vi "DHE_Aliases2.vi"(5 "expand reg":bool, 7 "action":T2(ring)=enum."find", 10 "name in":string) -> (1 "found?":bool, 2 "name out":string, 4 "register?":bool)   [LabVIEW 2016]
uses:
  private/vis/DHE_alias.ctl
  <vilib>/Utility/config.llb/Read Key (String).vi
  <vilib>/Utility/config.llb/NI_LVConfig.lvlib
panel:
  out "aliases":T1[](array[typedef])
  in  "alias":T1
  in  "error in (no error)":errorcluster
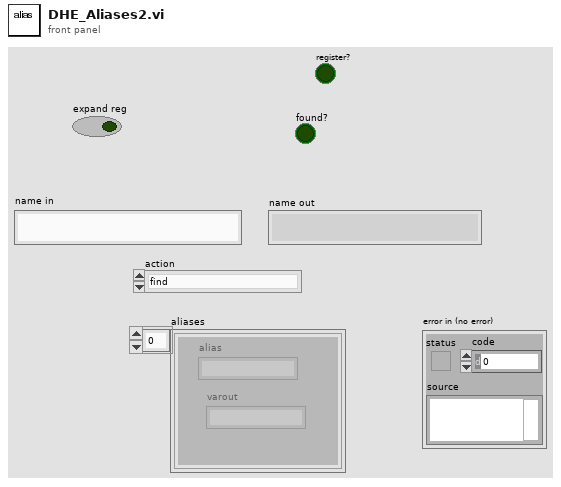
[diagram p1: front panel]
types:
  T1 = typedef "DHE_alias.ctl" = cluster{"alias":string, "varout":string}
  T2 = enum16{"read from file", "find", "get", "add", "delete", "clear "}
  T3 = typedef "NI_LVConfig.lvlib/Config Data RefNum.ctl" = refnum<k1>
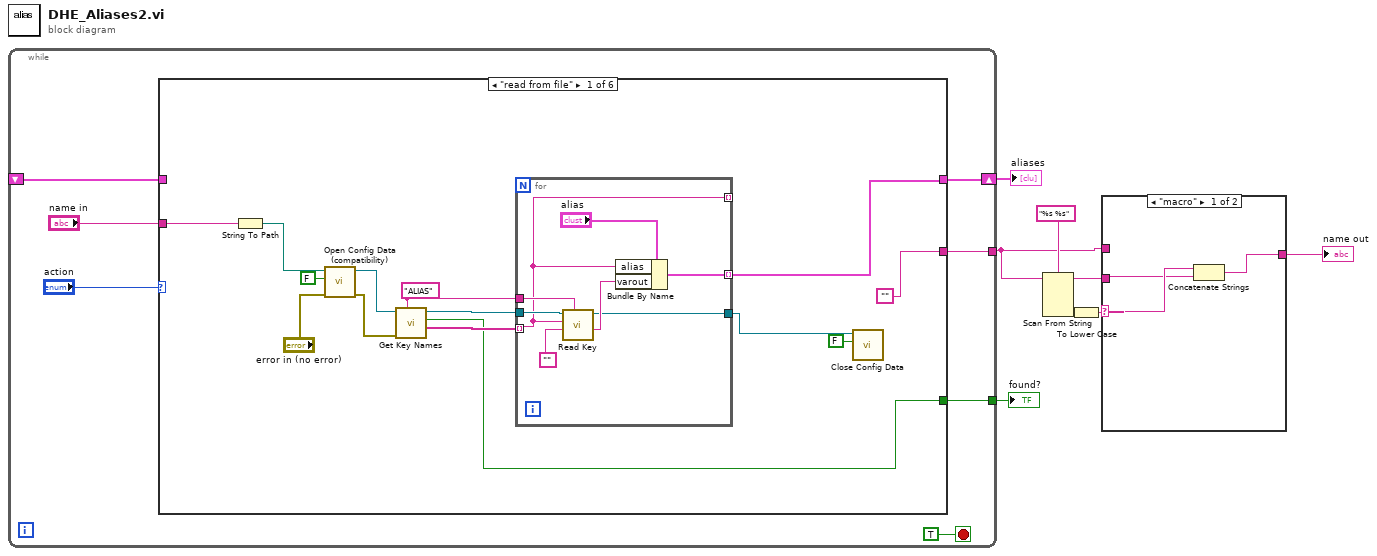
[diagram p0: block diagram]
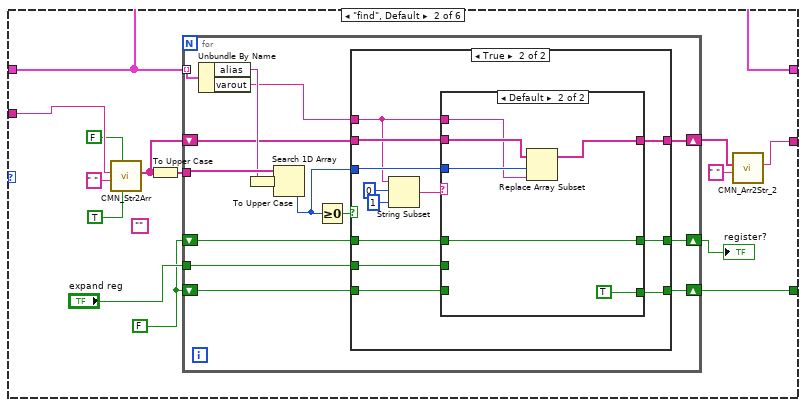
[diagram p3: hidden frame]
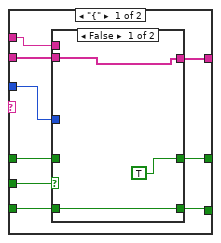
[diagram p5: hidden frame]
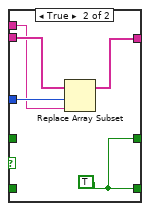
[diagram p6: hidden frame]
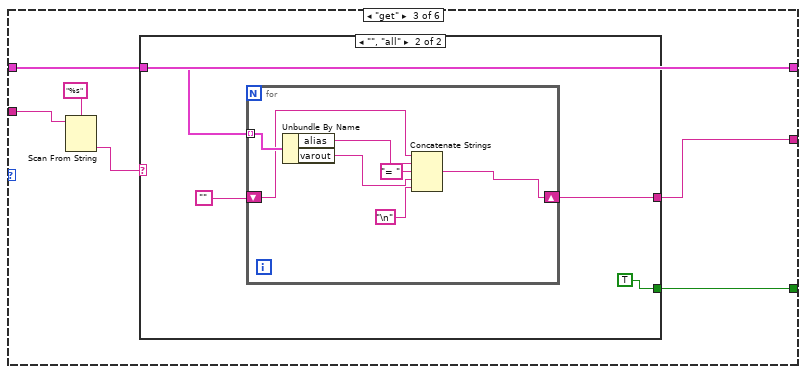
[diagram p7: hidden frame]
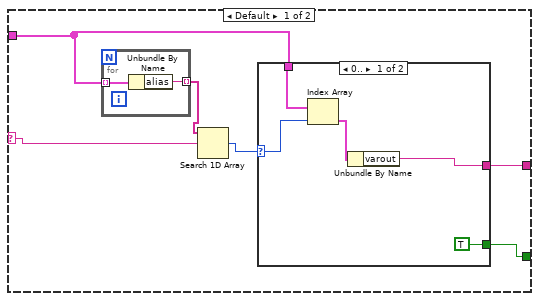
[diagram p8: hidden frame]
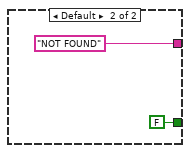
[diagram p9: hidden frame]
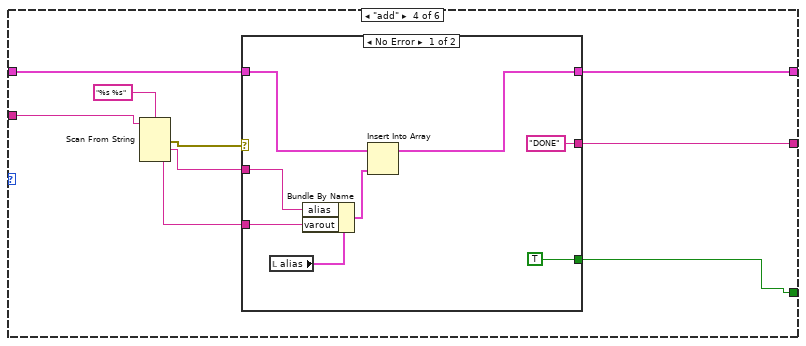
[diagram p10: hidden frame]
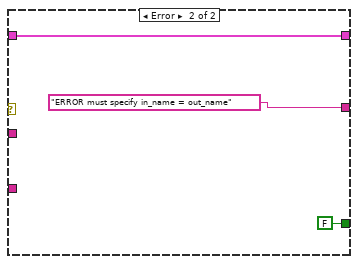
[diagram p11: hidden frame]
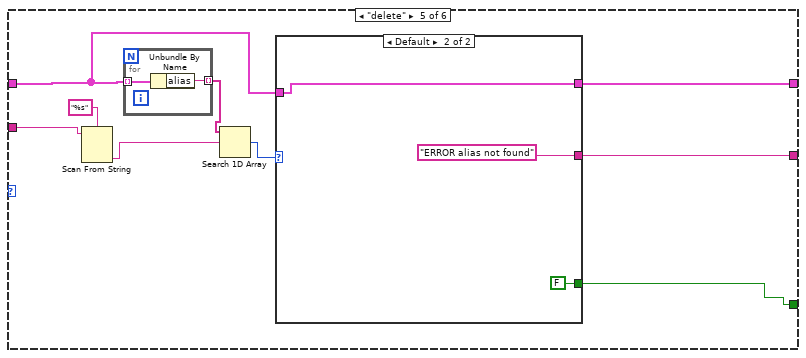
[diagram p12: hidden frame]
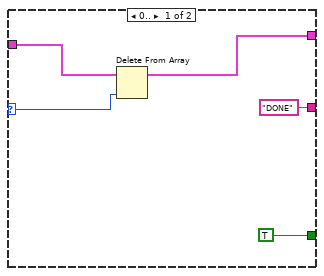
[diagram p13: hidden frame]
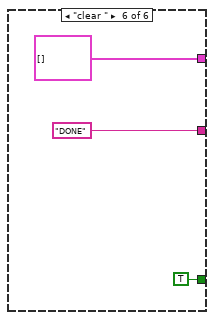
[diagram p14: hidden frame]
diagram:
  n1 = while {
    shift-right: [w14] -> w8
    shift-left: _ -> [w13]
    tunnel: [w10] -> w2
    tunnel: [w9] -> w7
    stop <- TRUE stop-if-true
    n2 = case shown="\"read from file\"" "action" {
      tunnel: [w23 w51 w109 w138 w162 T1[] []] -> w14
      tunnel: w13 -> [_ w51 w109 w144 w157 _]
      tunnel: "name in" -> [w21 w50 w107 w143 w164 _]
      tunnel: ["" w43 w108 w137 w161 "DONE" ("string out")] -> w10
      tunnel: [w16 w41 w104 w136 w156 TRUE ("section exists?")] -> w9
      frame "read from file" {
        w29 = "ALIAS" ("section")
        n3 = String To Path(string=w21) -> (path=w20:path)
        n4 = call <vilib>:"Open Config Data (compatibility).vi"("error in (no error)"="error in (no error)", "create file if necessary (T)"=FALSE, "configuration file path"=w20) -> ("error out"=w25:errorcluster, "refnum"=w24:T3)  [unwired: 6 in, 1 out]
        n5 = call <vilib>:"Get Key Names.vi"("section"=w29, "error in (no error)"=w25, "refnum"=w24) -> ("key names"=w28:string[], "section exists?"=w16:bool, "refnum out"=w27:T3)  [unwired: 6 out]
        n6 = for {
          tunnel: w27 -> [w37]
          tunnel: w29 -> [w36]
          tunnel: w28 -> [w31] mode=indexing
          tunnel: [w32] -> w23 mode=indexing
          tunnel: [w31] -> _ mode=indexing
          tunnel: [w30] -> w18
          n7 = call-poly <vilib>:"Read Key.vi"("section"=w36, "default value"="", "key"=w31, "refnum"=w37) -> ("value"=w33:string, "refnum out"=w30:T3)  [unwired: 2 in, 4 out]
          n8 = Bundle By Name(cluster="alias", "alias"=w31, "varout"=w33) -> (w32:T1)
        }
        n9 = call <vilib>:"Close Config Data.vi"("write file if changed (T)"=FALSE, "refnum"=w18) -> ()  [unwired: 8 in, 2 out]
      }
      frame "find", Default {
        w40 = FALSE
        (unwired) ""
        n10 = call "CMN_Str2Arr.vi"("trim"=TRUE, "strip quotation marks"=FALSE, "separator"=" ", "string in"=w50) -> ("Array out"=w46:string[])  [unwired: 7 in]
        n11 = To Upper Case(1:w46) -> (0:w38:string[])
        n12 = for {
          tunnel: w51 -> [w65] mode=indexing
          tunnel: w38 -> [w64]
          shift-right: [w58] -> w45
          shift-left: w46 -> [w61]
          tunnel: "expand reg" -> [w57]
          shift-right: [w55] -> w41
          shift-left: w40 -> [w56]
          shift-right: [w53] -> w39
          shift-left: w40 -> [w54]
          n13 = Unbundle By Name(w65) -> ("alias"=w63:string, "varout"=w59:string)
          n14 = To Upper Case(1:w63) -> (0:w52:string)
          n15 = Search 1D Array(1D array=w64, element=w52) -> (index of element=w60:i32)  [unwired: 1 in]
          n16 = Greater Or Equal To 0?(x=w60) -> (x >= 0?=w62:bool)
          n17 = case shown="True" w62 {
            tunnel: w61 -> [w68 w80]
            tunnel: w60 -> [_ w79]
            tunnel: w59 -> [_ w77]
            tunnel: [w68 w78] -> w58
            tunnel: w57 -> [_ w73]
            tunnel: w56 -> [w67 w72]
            tunnel: [w67 w71] -> w55
            tunnel: w54 -> [w66 w70]
            tunnel: [w66 w69] -> w53
            frame False {
            }
            frame True {
              n18 = String Subset(string=w77, offset (0)=0, length (rest)=1 ("length (rest)")) -> (substring=w74:string)
              n19 = case shown="Default" w74 {
                tunnel: w80 -> [w88 w103]
                tunnel: w79 -> [w87 w102]
                tunnel: w77 -> [w86 w101]
                tunnel: [w85 w100] -> w78
                tunnel: w73 -> [w89 _]
                tunnel: w72 -> [w84 _]
                tunnel: [w83 TRUE] -> w71
                tunnel: w70 -> [w82 w98]
                tunnel: [w81 w98] -> w69
                frame "{" {
                  n20 = case shown="False" w89 {
                    tunnel: w88 -> [w92 w96]
                    tunnel: w87 -> [_ w97]
                    tunnel: w86 -> [_ w95]
                    tunnel: [w92 w94] -> w85
                    tunnel: w84 -> [w91 _]
                    tunnel: [w91 w93] -> w83
                    tunnel: w82 -> [_ _]
                    tunnel: [TRUE w93] -> w81
                    frame False {
                    }
                    frame True {
                      w93 = TRUE
                      n21 = Replace Array Subset(array=w96, new element=w95, index=w97) -> (w94:string[])
                    }
                  }
                }
                frame Default {
                  n22 = Replace Array Subset(array=w103, new element=w101, index=w102) -> (w100:string[])
                }
              }
            }
          }
        }
        "register?" <- w39
        n23 = call "CMN_Arr2Str_2.vi"("separator"=" ", "Array in"=w45) -> ("string out"=w43:string)  [unwired: 9 in]
      }
      frame "get" {
        n24 = Scan From String(format string="%s", input string=w107) -> (output 1=w105:string)  [unwired: 3 in, 3 out]
        n25 = case shown="\"\", \"all\"" w105 {
          selector: w105 -> [w114 _]
          tunnel: w109 -> [w112 w128]
          tunnel: [w111 w126] -> w108
          tunnel: [w110 TRUE ("section exists?")] -> w104
          frame Default {
            n26 = for {
              tunnel: w112 -> [w124] mode=indexing
              tunnel: [w123] -> w115 mode=indexing
              n27 = Unbundle By Name(w124) -> ("alias"=w123:string)
            }
            n28 = Search 1D Array(1D array=w115, element=w114) -> (index of element=w113:i32)  [unwired: 1 in]
            n29 = case shown="0.." w113 {
              selector: w113 -> [w119 _]
              tunnel: w112 -> [w120 _]
              tunnel: [w117 "NOT FOUND" ("varout")] -> w111
              tunnel: [TRUE ("section exists?") FALSE ("section exists?")] -> w110
              frame 0.. {
                n30 = Index Array(array=w120, index=w119) -> (element=w118:T1)
                n31 = Unbundle By Name(w118) -> ("varout"=w117:string)
              }
              frame Default {
              }
            }
          }
          frame "", "all" {
            n32 = for {
              tunnel: w128 -> [w135] mode=indexing
              shift-right: [w129] -> w126
              shift-left: "" -> [w130]
              n33 = Unbundle By Name(w135) -> ("alias"=w134:string, "varout"=w132:string)
              n34 = Concatenate Strings(w130, w134, "= " ("string"), w132, "\n") -> (w129:string)
            }
          }
        }
      }
      frame "add" {
        n35 = Scan From String(format string="%s %s", input string=w143) -> (error out=w141:errorcluster, output 1=w140:string, output 2=w139:string)  [unwired: 4 in, 2 out]
        n36 = case shown="No Error" w141 {
          tunnel: w144 -> [w152 w155]
          tunnel: w140 -> [w150 _]
          tunnel: w139 -> [w149 _]
          tunnel: [w147 w155] -> w138
          tunnel: ["DONE" ("string out") "ERROR must specify in_name = out_name" ("string out")] -> w137
          tunnel: [TRUE ("section exists?") FALSE ("section exists?")] -> w136
          frame No Error {
            n37 = local read "alias"() -> (w151:T1)
            n38 = Bundle By Name(cluster=w151, "alias"=w150, "varout"=w149) -> (w148:T1)
            n39 = Insert Into Array(array=w152, new element=w148) -> (w147:T1[])  [unwired: 1 in]
          }
          frame Error {
          }
        }
      }
      frame "delete" {
        n40 = Scan From String(format string="%s", input string=w164) -> (output 1=w159:string)  [unwired: 3 in, 3 out]
        n41 = for {
          tunnel: w157 -> [w166] mode=indexing
          tunnel: [w165] -> w160 mode=indexing
          n42 = Unbundle By Name(w166) -> ("alias"=w165:string)
        }
        n43 = Search 1D Array(1D array=w160, element=w159) -> (index of element=w158:i32)  [unwired: 1 in]
        n44 = case shown="Default" w158 {
          selector: w158 -> [w169 _]
          tunnel: [w168 w173] -> w162
          tunnel: ["DONE" ("string out") "ERROR alias not found" ("string out")] -> w161
          tunnel: w157 -> [w170 w173]
          tunnel: [TRUE ("section exists?") FALSE ("section exists?")] -> w156
          frame 0.. {
            n45 = Delete From Array(array=w170, index=w169) -> (array with subset deleted=w168:T1[])  [unwired: 1 in, 1 out]
          }
          frame Default {
          }
        }
      }
      frame "clear " {
      }
    }
  }
  "aliases" <- w8
  "found?" <- w7
  n46 = Scan From String(format string="%s %s", input string=w2) -> (remaining string=w4:string, output 2=w5:string)  [unwired: 5 in, 2 out]
  n47 = To Lower Case(string=w5) -> (all lower case string=w3:string)
  n48 = case shown="\"macro\"" w3 {
    selector: w3 -> [w180 _]
    tunnel: w4 -> [w179 _]
    tunnel: w2 -> [_ w181]
    tunnel: [w178 w181] -> w1
    frame "macro" {
      n49 = Concatenate Strings(w180, w179) -> (w178:string)
    }
    frame Default {
    }
  }
  "name out" <- w1
